vi "Run Remote Instrument Script.vi"(7 "Script Source Code":string, 8 "error in (no error)":errorcluster, 9 "Script Name (Nil)":string="Nil", 10 "Instrument ID":string, 11 "VISA resource name":refnum<visa-resource-name>) -> (0 "error out":errorcluster, 3 "VISA resource name out":refnum<visa-resource-name>)   [LabVIEW 2019, in "Keithley 2600 Series.lvlib"]
doc: "Loads and runs a script on a remote TSP-enabled instrument.\n\n<b>Note:</b>\nThis VI is not available on the Models 2604B, 2614B, and 2634B."
uses:
  Keithley 2600 Series.lvlib
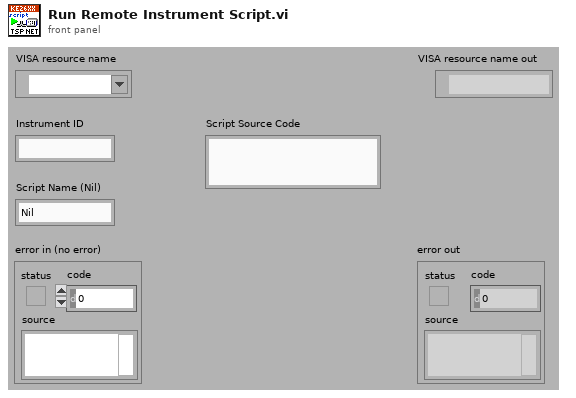
[diagram p1: front panel]
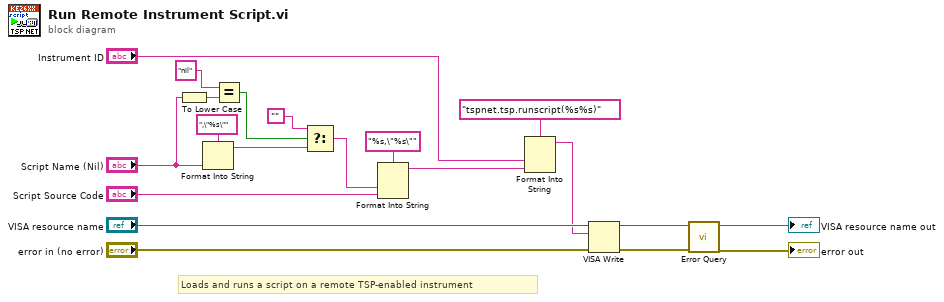
[diagram p0: block diagram]
diagram:
  # "Loads and runs a script on a remote TSP-enabled instrument"
  n1 = To Lower Case(string="Script Name (Nil)") -> (all lower case string=w2:string)
  n2 = Format Into String(format string=",\"%s\"", "Script Name (Nil)") -> (resulting string=w8:string)  [unwired: 2 in, 1 out]
  n3 = Equal?(x="nil", y=w2) -> (x = y?=w11:bool)
  n4 = Select(t="", s=w11, f=w8) -> (s? t:f=w6:string)
  n5 = Format Into String(format string="%s,\"%s\"", w6, "Script Source Code") -> (resulting string=w4:string)  [unwired: 2 in, 1 out]
  n6 = Format Into String(format string="tspnet.tsp.runscript(%s%s)", "Instrument ID", w4) -> (resulting string=w3:string)  [unwired: 2 in, 1 out]
  n7 = VISA Write(VISA resource name="VISA resource name", write buffer=w3, error in (no error)="error in (no error)") -> (VISA resource name out=w17:refnum<visa-resource-name>, error out=w16:errorcluster)  [unwired: 1 out]
  n8 = call "Error Query.vi"("error in (no error)"=w16, "VISA resource name"=w17) -> ("error out"=→"error out":errorcluster, "VISA resource name out"=→"VISA resource name out":refnum<visa-resource-name>)  [unwired: 6 in, 2 out]
